vi "Measurement.vi"(8 "error in (no error)":errorcluster, 11 "Experiment2D in":refnum<class "Experiment2D.lvclass">) -> (0 "error out":errorcluster, 1 "Finish?":bool, 2 "Result":dbl, 3 "Experiment2D out":refnum<class "Experiment2D.lvclass">)   [LabVIEW 2014, in "Experiment2D.lvclass"]
uses:
  Experiment2D.lvclass
  Measurement/Measurement2D/Measurement2D.lvclass
  Data/Data2D/Data2D.lvclass
panel:
  out "Current Value":dbl
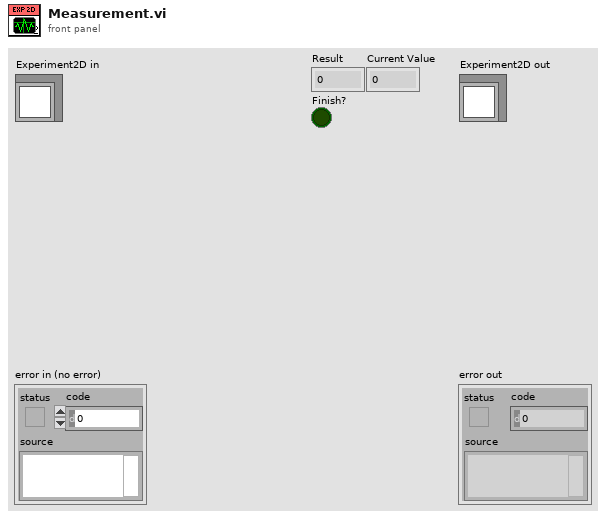
[diagram p1: front panel]
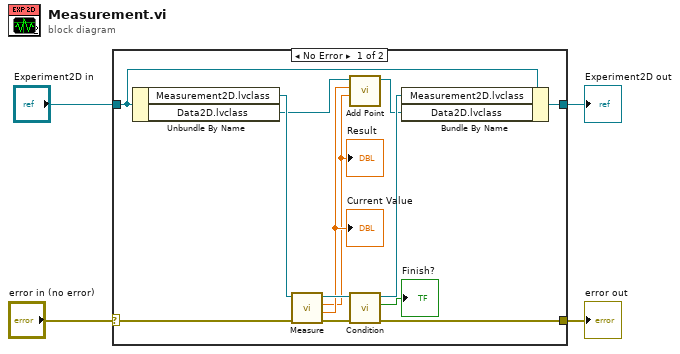
[diagram p0: block diagram]
diagram:
  n1 = case shown="No Error" "error in (no error)" {
    selector: "error in (no error)" -> [w11 w19]
    tunnel: [w9 w19] -> w3
    tunnel: [w12 w18] -> w1
    tunnel: "Experiment2D in" -> [w14 w18]
    frame No Error {
      n2 = Unbundle By Name(w14) -> ("Measurement2D.lvclass"=w17:refnum<class "Measurement2D.lvclass">, "Data2D.lvclass"=w8:refnum<class "Data2D.lvclass">)
      n3 = call-dynamic "Measure.vi"("error in (no error)"=w11, "Measurement2D in"=w17) -> ("error out"=w10:errorcluster, "Current Value"=w7:dbl, "Result"=w6:dbl, "Measurement2D out"=w16:refnum<class "Measurement2D.lvclass">)  [unwired: 6 in]
      "Result" <- w6
      "Current Value" <- w7
      n4 = call-dynamic "Add Point.vi"("Y"=w6, "X"=w7, "Data2D in"=w8) -> ("Data2D out"=w5:refnum<class "Data2D.lvclass">)  [unwired: 7 in, 1 out]
      n5 = call-dynamic "Condition.vi"("error in (no error)"=w10, "Measurement2D in"=w16) -> ("error out"=w9:errorcluster, "Finish?"=→"Finish?":bool, "Measurement2D out"=w13:refnum<class "Measurement2D.lvclass">)  [unwired: 7 in]
      n6 = Bundle By Name(cluster=w14, "Measurement2D.lvclass"=w13, "Data2D.lvclass"=w5) -> (w12:refnum<class "Experiment2D.lvclass">)
    }
    frame Error {
    }
  }
  "error out" <- w3
  "Experiment2D out" <- w1
